vi "Demo.vi"() -> ()   [LabVIEW 2009]
uses:
  XControl/XMenuBar.xctl
  XControl/CMenu/CMenu.lvclass
panel:
  in  "Exit":bool
  out "User Selected Item Tag:":string
  in  "XMenuBar":refnum<class "CMenu.lvclass">(xcontrol)
  # "Demo XMenu V1.0"
  # "Demo Instruction:\n1) Drag \"Xmenu\" Control to your GUI;\n2) Righ click the control and select \"Edit Xmenu Items\";\n3) Use \"Menu Editor\" custom menu for your application;\n4) Run and play!"
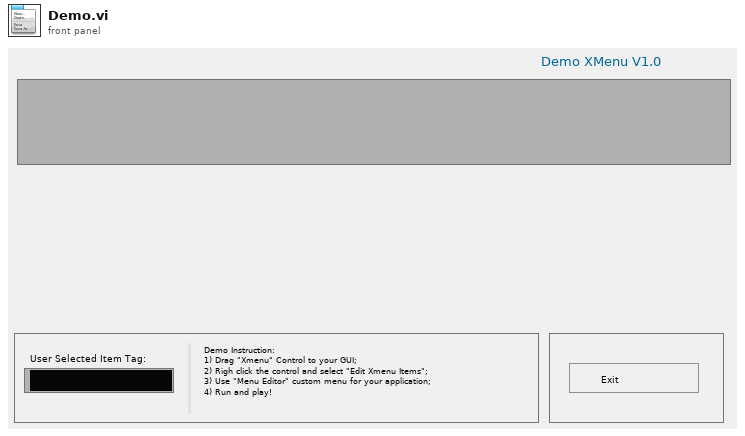
[diagram p1: front panel]
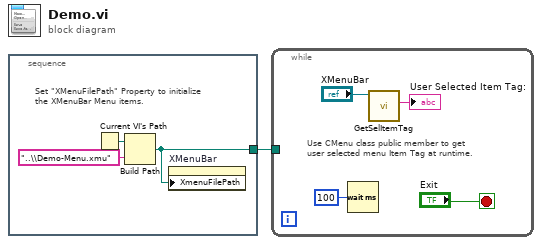
[diagram p0: block diagram]
diagram:
  n1 = stacked-sequence {
    tunnel: [w2] -> w1
    frame #0 {
      # "Set \"XMenuFilePath\" Property to initialize\nthe XMenuBar Menu items."
      n2 = Current VI's Path() -> (path=w4:path)
      n3 = Build Path(base path=w4, name or relative path="..\\Demo-Menu.xmu") -> (appended path=w2:path)
      n4 = property on="XMenuBar" class="XMenuBar (strict)"("XmenuFilePath"=w2) -> ()  [unwired: 2 in, 2 out]
    }
  }
  n5 = while {
    tunnel: w1 -> [_]
    stop <- "Exit" stop-if-true
    # "Use CMenu class public member to get \nuser selected menu Item Tag at runtime."
    n6 = Wait (ms)(milliseconds to wait=u32 100) -> ()  [unwired: 1 out]
    n7 = call "GetSelItemTag.vi"("CMenu in"="XMenuBar") -> ("SelItemTag"=→"User Selected Item Tag:":string)  [unwired: 8 in, 2 out]
  }
